vi "command add sync in action.vi"(8 "error in (no error)":errorcluster, 10 "the_command_add_sync_in_action":T1, 11 "id":i32) -> (0 "error out":errorcluster, 3 "function return":i32)   [LabVIEW 2012, in "libximc.lvlib"]
doc: "result_t XIMC_API command_add_sync_in_action (device_t id, const command_add_sync_in_action_t* the_command_add_sync_in_action);"
uses:
  libximc.lvlib
  libximc.dll
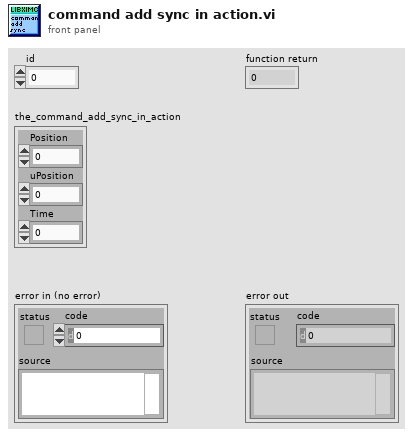
[diagram p1: front panel]
types:
  T1 = cluster{"Position":i32, "uPosition":i32, "Time":u32}
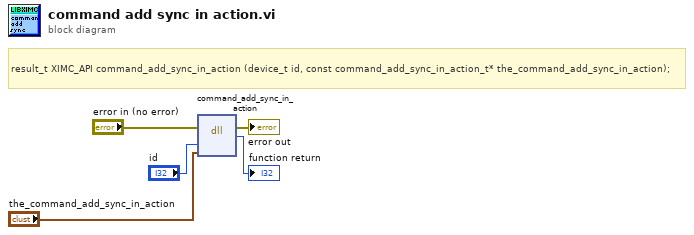
[diagram p0: block diagram]
diagram:
  # "result_t XIMC_API command_add_sync_in_action (device_t id, const command_add_sync_in_action_t* the_command_add_sync_in_action);"
  n1 = dll-call lib="E:/labview-2.12.1-Labview_12.0/ximcLVx32/libximc.*" fn="command_add_sync_in_action"(error in="error in (no error)", "id"="id", "the_command_add_sync_in_action"="the_command_add_sync_in_action") -> (error out=→"error out":errorcluster, →"function return":i32)  [unwired: 4 in, 1 out]
